vi "Int64 Destroy.vi"(8 "error in (no error)":errorcluster, 11 "Int64 DVR in":refnum<data-value>) -> (0 "error out":errorcluster)   [LabVIEW 2015, in "MDSplus.lvlib"]
uses:
  <vilib>/MDSplus/Library/MDSplus.lvlib
  <vilib>/MDSplus/Classes/Data_Class/Scalar_Class/Int64_Class/Int64.lvclass
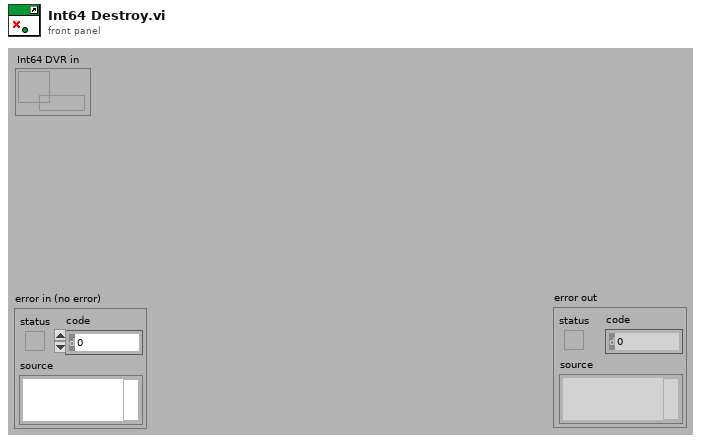
[diagram p1: front panel]
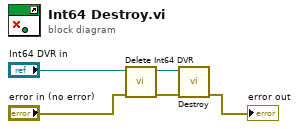
[diagram p0: block diagram]
diagram:
  n1 = call <vilib>:"Delete Int64 DVR.vi"("error in (no error)"="error in (no error)", "Int64 DVR in"="Int64 DVR in") -> ("error out"=w2:errorcluster, "Int64 out"=w3:refnum<class "Int64.lvclass">)  [unwired: 8 in]
  n2 = call-dynamic "Destroy.vi"("error in (no error)"=w2, "Int64 in"=w3) -> ("error out"=→"error out":errorcluster)  [unwired: 9 in]
